vi "read37(measurement).vi"(0 "VISA资源名称":refnum<visa-resource-name>, 5 "文件（使用对话框）":path, 7 "连接":bool) -> (4 "本次":string)   [LabVIEW 2017]
uses:
  <vilib>/Instr/_visa.llb/VISA Configure Serial Port (Instr).vi
  <vilib>/addons/Tools/Unicode/UTF8 Tools.lvlib
panel:
  out "错误输出 2":errorcluster caption="错误输出"
  in  "?":enum32{"CONTROL", "选项卡 2"}(tab)
  in  "增益选择":u16(ring) items=["±6.144V", "±4.096V", "±2.048V", "±1.024V", "±0.512V", "±0.256V"]
  in  "连接方式":u16(ring) items=["Serial", "WiFi", "Dual"]
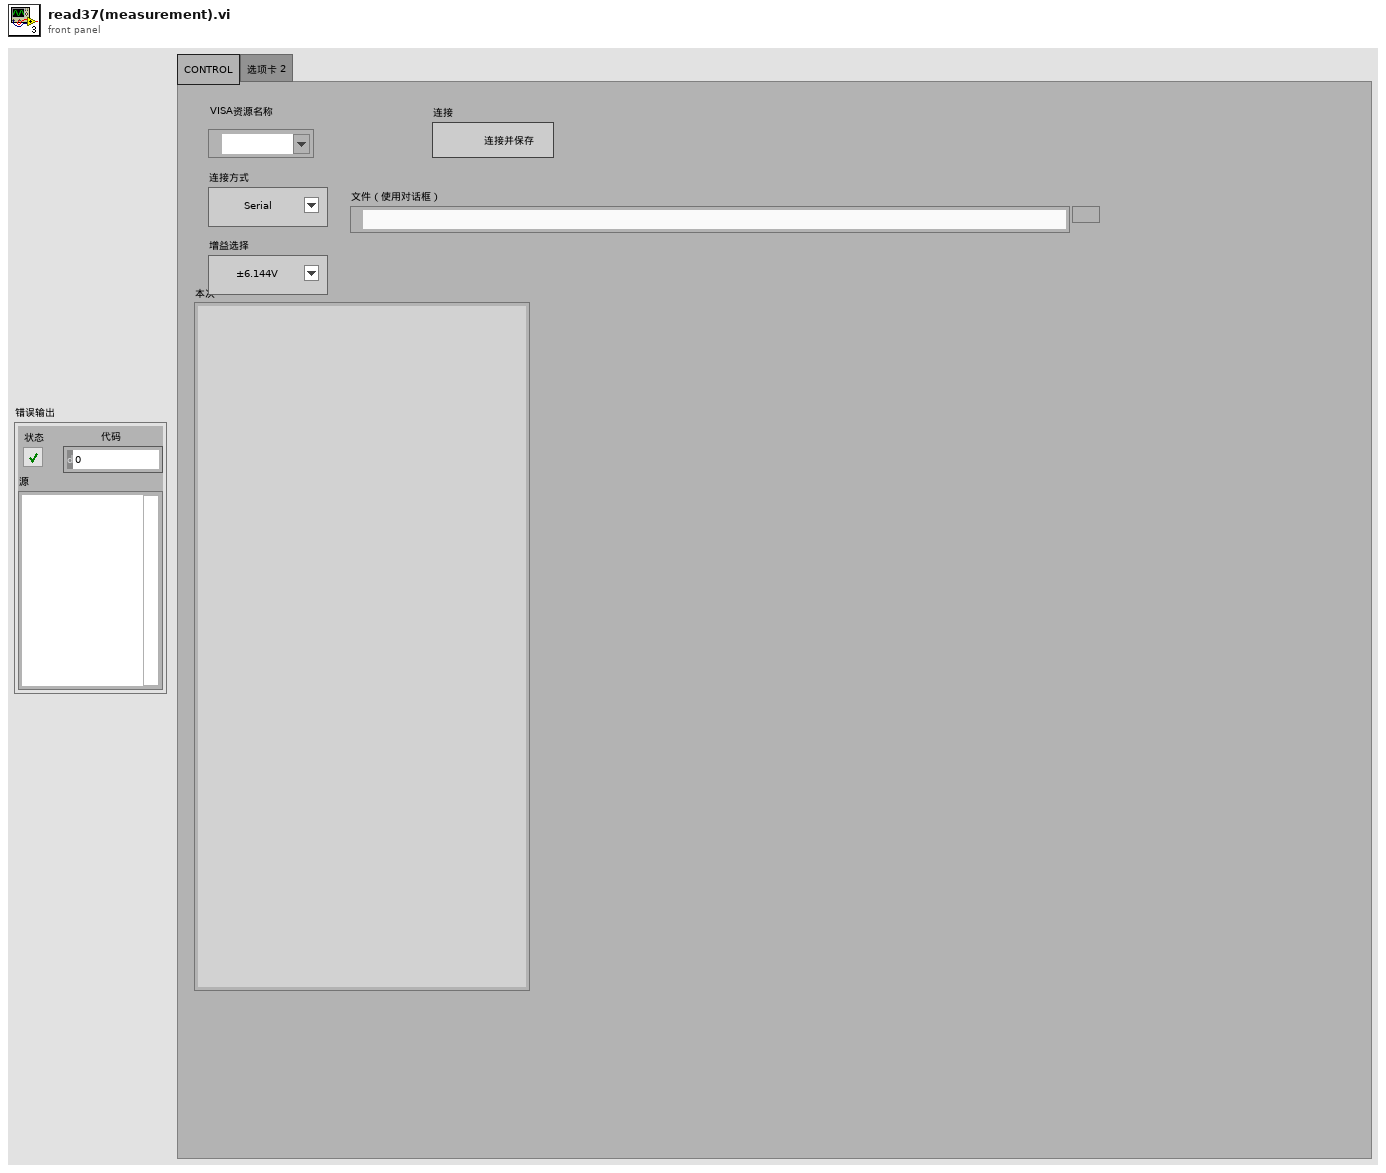
[diagram p1: front panel]
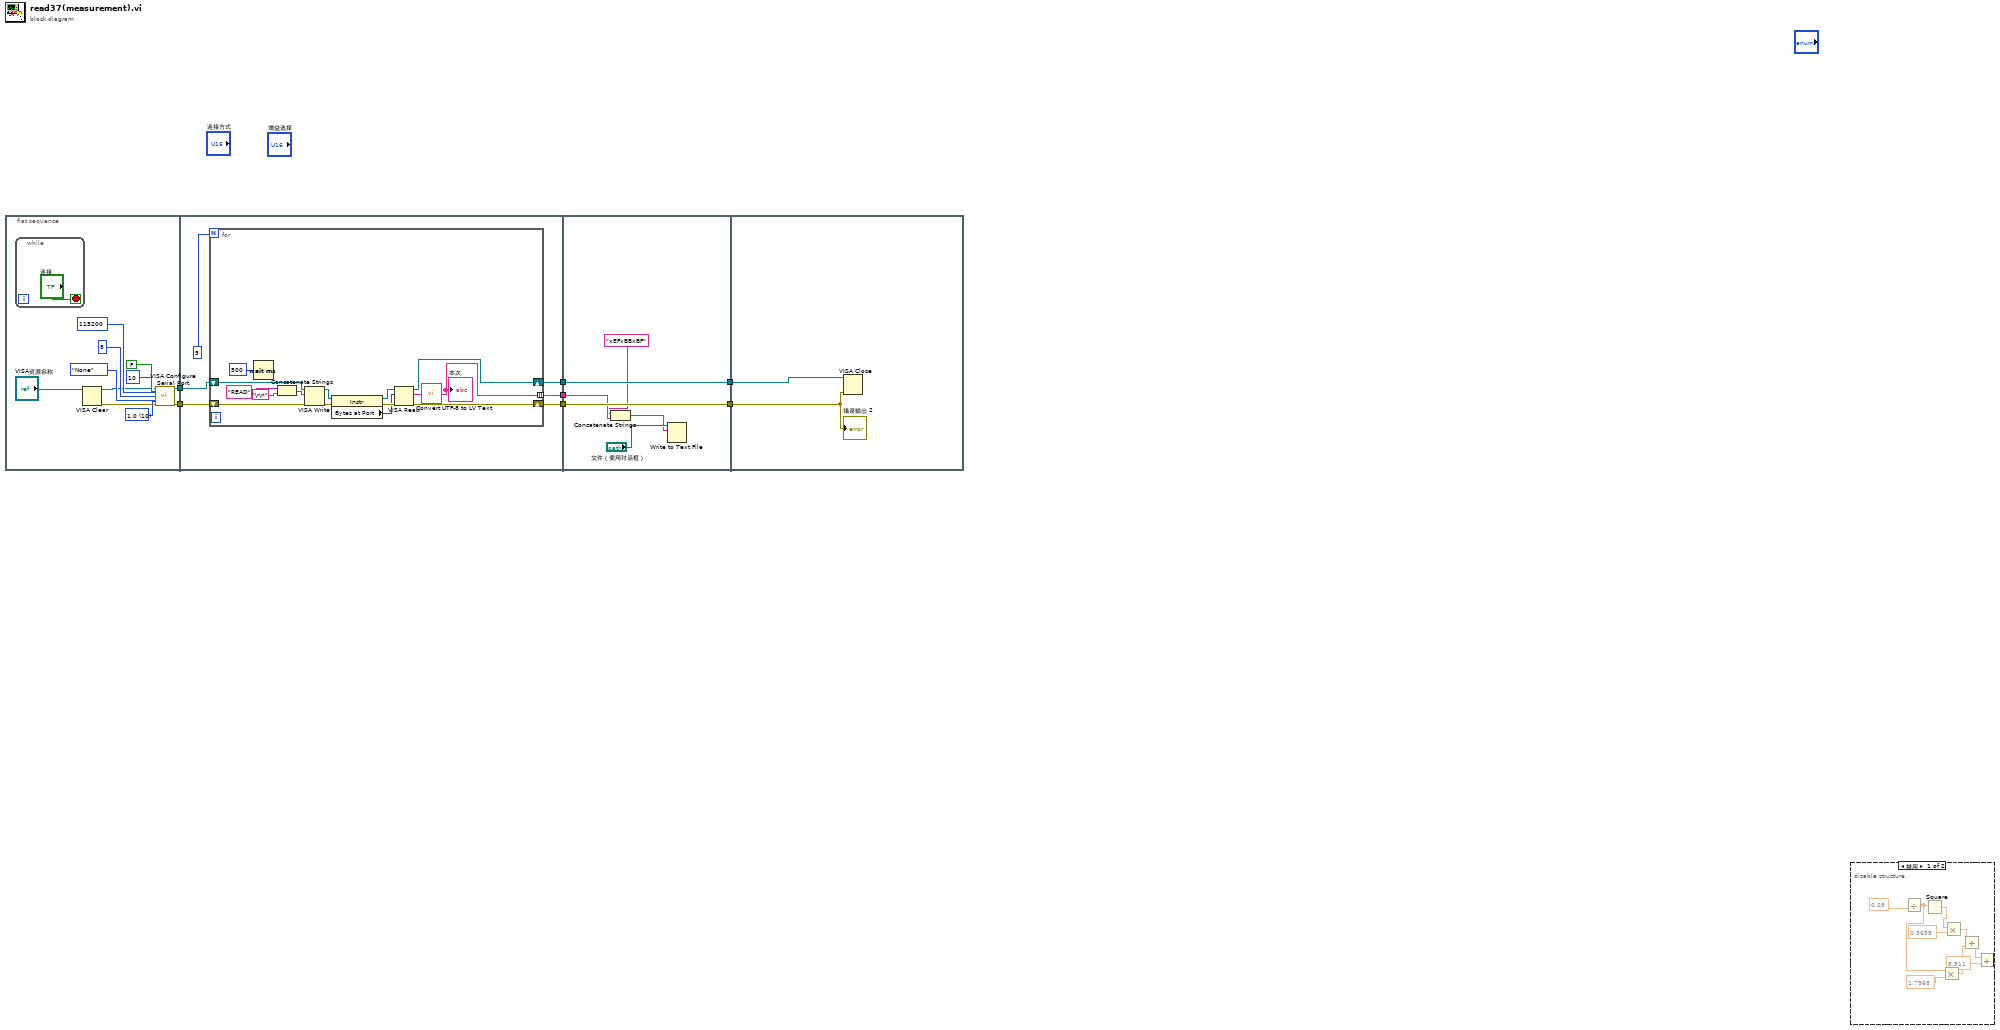
[diagram p0: block diagram]
diagram:
  n1 = flat-sequence {
    tunnel: [w10] -> w7
    tunnel: [w9] -> w6
    tunnel: w7 -> [w25]
    tunnel: w6 -> [w24]
    tunnel: [w23] -> w5
    tunnel: [w22] -> w3
    tunnel: [w20] -> w1
    tunnel: w5 -> [w46]
    tunnel: [w46] -> w4
    tunnel: w3 -> [w45]
    tunnel: [w45] -> w2
    tunnel: w1 -> [w43]
    tunnel: w4 -> [w48]
    tunnel: w2 -> [w47]
    frame #0 {
      w17 = u16 10 items=["1.0"=10, "1.5"=15, "2.0"=20] ("stop bits (10: 1 bit)")
      n2 = while {
        stop <- "连接" stop-if-true
      }
      n3 = VISA Clear(VISA resource name="VISA资源名称") -> (VISA resource name out=w13:refnum<visa-resource-name>, error out=w12:errorcluster)  [unwired: 1 in]
      n4 = call-poly "VISA Configure Serial Port"("VISA resource name"=w13, "termination char\n(0xA = '\\n' = LF)"=u8 10 ("termination char\n(0xA = '\\n' = LF)"), "Enable Termination\nChar (T)"=FALSE ("Enable Termination\nChar (T)"), "baud rate (9600)"=u32 115200, "data bits (8)"=u16 8, "parity (0:none)"=enum16{"None", "Odd", "Even", "Mark", "Space"}."None", "error in (no error)"=w12, "stop bits (10: 1 bit)"=w17) -> ("VISA resource name out"=w9:refnum<visa-resource-name>, "error out"=w10:errorcluster)  [unwired: 6 in]
    }
    frame #1 {
      n5 = for {
        N: 5 -> [_]
        shift-right: [w37] -> w22
        shift-left: w25 -> [w40]
        shift-right: [w38] -> w23
        shift-left: w24 -> [w39]
        tunnel: [w26] -> w20 mode=indexing
        n6 = Wait (ms)(milliseconds to wait=u32 500 ("等待时间（毫秒）")) -> ()  [unwired: 1 out]
        n7 = Concatenate Strings("READ" ("字符串"), "\r\n") -> (w36:string)
        n8 = VISA Write(VISA resource name=w39, write buffer=w36, error in (no error)=w40) -> (VISA resource name out=w35:refnum<visa-resource-name>, error out=w34:errorcluster)  [unwired: 1 out]
        n9 = property class="Instr"(reference=w35, error in=w34) -> (reference out=w32:refnum<visa-resource-name>, error out=w31:errorcluster, "Bytes at Port"=w30:u32)
        n10 = VISA Read(VISA resource name=w32, byte count=w30, error in (no error)=w31) -> (VISA resource name out=w38:refnum<visa-resource-name>, read buffer=w27:string, error out=w37:errorcluster)  [unwired: 1 out]
        n11 = call <vilib>:"Convert UTF-8 to LV Text.vi"("UTF-8 Text"=w27) -> ("LV Text"=w26:string)  [unwired: 13 in, 1 out]
        "本次" <- w26
      }
    }
    frame #2 {
      n12 = Concatenate Strings("xEFxBBxBF", w43) -> (w42:string)
      n13 = Write to Text File(file (use dialog)="文件（使用对话框）", text=w42) -> ()  [unwired: 2 in, 3 out]
    }
    frame #3 {
      n14 = VISA Close(VISA resource name=w48, error in (no error)=w47) -> ()  [unwired: 1 out]
      "错误输出 2" <- w47
    }
  }
  n15 = disable-structure shown="禁用" {
    frame Disabled {
      n16 = Divide(y=0.05) -> (x/y=w53:dbl)  [unwired: 1 in]
      n17 = Square(x=w53) -> (x^2=w56:dbl)
      n18 = Multiply(x=w53, y=1.7968) -> (x*y=w51:dbl)
      n19 = Multiply(x=w56, y=0.3658) -> (x*y=w54:dbl)
      n20 = Add(x=w54, y=w51) -> (x+y=w50:dbl)
      n21 = Add(x=w50, y=8.511) -> ()  [unwired: 1 out]
    }
    frame Enabled {
    }
  }
